vi "donneespointagetofinance.vi"() -> (0 "Date_fin":timestamp[](array[timestamp]), 1 "Date_debut":timestamp[](array[timestamp]))   [LabVIEW 2024]
uses:
  <vilib>/drjdpowell/SQLite Library/SQL Connection/Open (string).vi
  <vilib>/drjdpowell/SQLite Library/SQL Connection/Execute SQL.vi
  <vilib>/drjdpowell/SQLite Library/SQL Connection/Connection.lvclass
  <vilib>/drjdpowell/SQLite Library/SQLite.lvlib
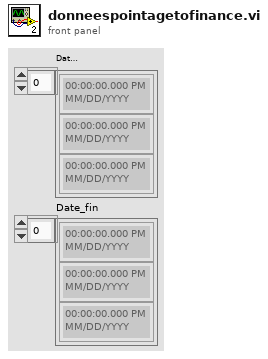
[diagram p1: front panel]
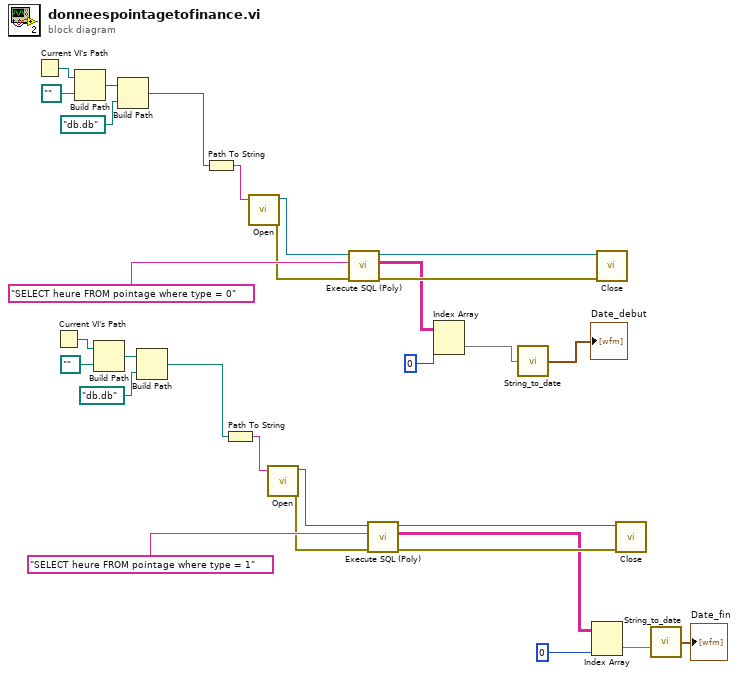
[diagram p0: block diagram]
diagram:
  n1 = Current VI's Path() -> (path=w25:path)
  n2 = Current VI's Path() -> (path=w14:path)
  n3 = Build Path(base path=w25, name or relative path=path "..") -> (appended path=w22:path)
  n4 = Build Path(base path=w14, name or relative path=path "..") -> (appended path=w11:path)
  n5 = Build Path(base path=w22, name or relative path=path "db.db" ("Filename")) -> (appended path=w21:path)
  n6 = Build Path(base path=w11, name or relative path=path "db.db" ("Filename")) -> (appended path=w10:path)
  n7 = Path To String(path=w21) -> (string=w20:string)
  n8 = Path To String(path=w10) -> (string=w9:string)
  n9 = call-poly <vilib>:"Open.vi"("db file"=w20) -> ("error out"=w26:errorcluster, "SQLite Connection"=w27:refnum<class "Connection.lvclass">)  [unwired: 9 in]
  n10 = call-poly <vilib>:"Open.vi"("db file"=w9) -> ("error out"=w15:errorcluster, "SQLite Connection"=w16:refnum<class "Connection.lvclass">)  [unwired: 9 in]
  n11 = call-poly <vilib>:"Execute SQL (Poly).vi"("error in (no error)"=w26, "SQL"="SELECT heure FROM pointage where type = 0", "SQLite Connection in"=w27) -> ("error out"=w29:errorcluster, "Result Set"=w8:string[][], "SQLite Connection"=w30:refnum<class "Connection.lvclass">)  [unwired: 5 in, 1 out]
  n12 = call-poly <vilib>:"Execute SQL (Poly).vi"("error in (no error)"=w15, "SQL"="SELECT heure FROM pointage where type = 1", "SQLite Connection in"=w16) -> ("error out"=w18:errorcluster, "Result Set"=w5:string[][], "SQLite Connection"=w19:refnum<class "Connection.lvclass">)  [unwired: 5 in, 1 out]
  n13 = Index Array(array=w8, index (col)=0) -> (element=w4:string[])  [unwired: 1 in]
  n14 = call "String_to_date.vi"("String"=w4) -> ("Date"=→"Date_debut":timestamp[])
  n15 = Index Array(array=w5, index (col)=0) -> (element=w2:string[])  [unwired: 1 in]
  n16 = call-dynamic "Close.vi"("error in (no error)"=w29, "SQLite Connection in"=w30) -> ()  [unwired: 9 in, 1 out]
  n17 = call-dynamic "Close.vi"("error in (no error)"=w18, "SQLite Connection in"=w19) -> ()  [unwired: 9 in, 1 out]
  n18 = call "String_to_date.vi"("String"=w2) -> ("Date"=→"Date_fin":timestamp[])
